vi "DelayR.vi"(2 "R":bool, 3 "DelayOff":u32, 4 "DelayOn":u32, 5 "In":bool) -> (0 "t ms":u32, 1 "Out":bool)   [LabVIEW 2019, in "Timers.lvlib"]
uses:
  Timers.lvlib
  Logik/Logik.lvlib
  Trigers/Triggers.lvlib
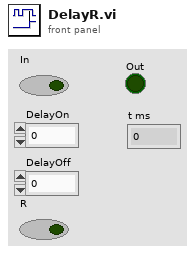
[diagram p1: front panel]
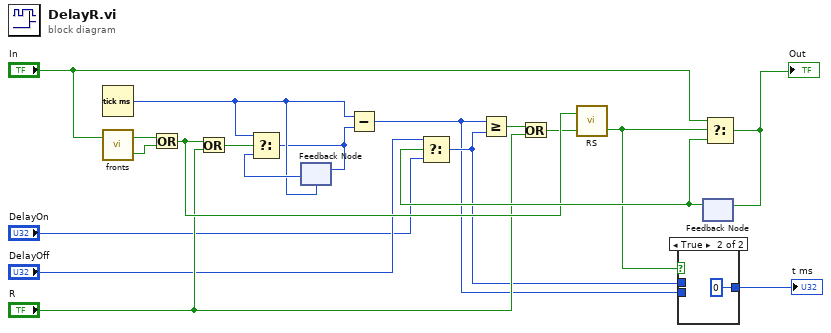
[diagram p0: block diagram]
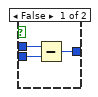
[diagram p2: hidden frame]
diagram:
  n1 = Tick Count (ms)() -> (millisecond timer value=w18:u32)
  n2 = call "fronts.vi"("in"="In") -> ("fall"=w14:bool, "raise"=w15:bool)  [unwired: 1 in]
  n3 = Or(x=w15, y=w14) -> (x .or. y?=w10:bool)
  n4 = Or(x=w10, y="R") -> (x .or. y?=w11:bool)
  n5 = feedback #1(w18) -> (w19:u32)
  n6 = Select(t=w18, s=w11, f=w19) -> (s? t:f=w13:u32)
  n7 = feedback-in #1(w13) -> ()
  n8 = Subtract(x=w18, y=w13) -> (x-y=w4:u32)
  n9 = feedback #2() -> (w12:bool)  [unwired: 1 in]
  n10 = Select(t="DelayOff", s=w12, f="DelayOn") -> (s? t:f=w5:u32)
  n11 = Greater Or Equal?(x=w4, y=w5) -> (x >= y?=w8:bool)
  n12 = Or(x=w8, y="R") -> (x .or. y?=w7:bool)
  n13 = call "RS.vi"("R"=w7, "S"=w10) -> ("~Q"=w6:bool)  [unwired: 1 out]
  n14 = case shown="True" w6 {
    tunnel: w5 -> [w22 _]
    tunnel: w4 -> [w21 _]
    tunnel: [w20 u32 0] -> w3
    frame False {
      n15 = Subtract(x=w22, y=w21) -> (x-y=w20:u32)
    }
    frame True {
    }
  }
  "t ms" <- w3
  n16 = Select(t="In", s=w6, f=w12) -> (s? t:f=w16:bool)
  "Out" <- w16
  n17 = feedback-in #2(w16) -> ()
